vi "output_FPGA.vi"() -> ()   [LabVIEW 2021]
uses:
  <vilib>/Platform/TimedLoop/XDataNode/timing_clust.ctl
  <vilib>/Platform/TimedLoop/XDataNode/nitl_modes.ctl
  <vilib>/Platform/TimedLoop/XDataNode/wakeup.ctl
  <vilib>/rvi/Emulation/niFpgaGetClockAttributes.vi
  <vilib>/rvi/Emulation/niFpgaSctlEmulationGetInTimedLoop.vi
  <vilib>/rvi/Emulation/niFpgaEmulationReportErrorSimple.vi
  <vilib>/rvi/Emulation/niFpgaProcessEmulError.vi
  <vilib>/rvi/interface/RandomDataEmulation/niFpgaRandomDataHandleErrors.vi
  <vilib>/rvi/Emulation/niFpgaCriticalErrorInLSC.vi
  <vilib>/rvi/eio/common/nirviEmuTemplateMethod_errors.vi
  <vilib>/rvi/DataTransferAndStorage/Container/XNode/niFpgaContainer.xnode
  <vilib>/rvi/interface/RandomDataEmulation/nirviRandomDataFpgaReadWriteTemplate.vi
  <vilib>/eio/EIONode/EIONode.xnode
  <vilib>/Platform/TimedLoop/XDataNode/XDataNode.xnode
  <vilib>/Platform/TimedLoop/XDataNode/XDNodeRunTimeDep.lvlib
panel:
  out "Connector 1 DIO Port 0":u8
  out "Connector 1 DIO Port 1":u8
  out "Connector 1 DIO Port 2":u8
  out "Connector 1 DIO Port 3":u8
  in  "Connector 2 DIO Port 0":u8
  in  "Connector 2 DIO Port 1":u8
  out "AO: Actual Loop Rate(ticks)":u32
  in  "AO 0":i16
  in  "AO 1":i16
  in  "AO 2":i16
  in  "AO 3":i16
  in  "AO 4":i16
  in  "AO 5":i16
  in  "AO 6":i16
  in  "AO 7":i16
  in  "AO Loop Timer(Ticks)":u32
  out "AO Buffer Underflow?":bool
  in  "AO Buffer Enable":u8 format="%08b"
  in  "AO Enable":bool
  # "Analog Output"
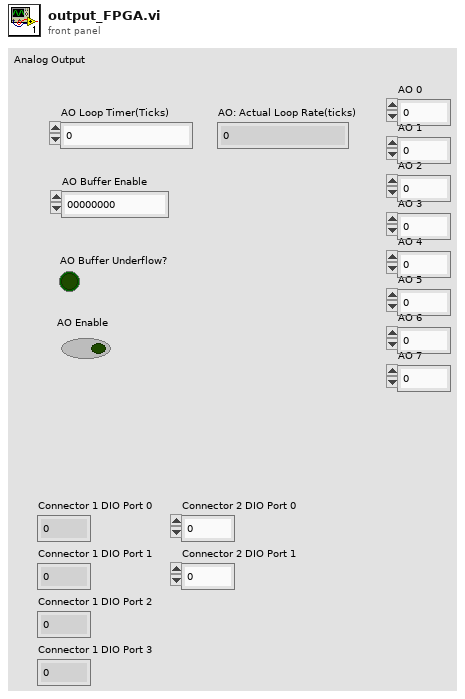
[diagram p1: front panel]
types:
  T1 = typedef "XDNodeRunTimeDep.lvlib/timing_clust.ctl" = cluster{"Expected End [f-1]":u64, "Actual End [f-1]":u64, "Finished Late? [f-1]":bool, "Expected End [i-1]":u64, "Actual End [i-1]":u64, "Finished Late? [i-1]":bool, "Expected Start [i]":u64, "Actual Start [i]":u64, "Expected Start [f]":u64, "Actual Start [f]":u64, "Source Name":string, "Structure Name":string, "Period":i64, "Deadline":i64, "Offset":i64, "Start":i64, "Priority":i32, "Timeout":i32, "Mode":T2, "Wakeup Reason":T3, "Error":errorcluster, "Source Type":string, "Secondary Source Type":string, "Global End Time":u64, "Global Start Time":u64, "Frame Duration":u64, "Iteration Duration":u64, "Assigned CPU":i32, "I/O Scan Engine Mode":u32}
  T2 = typedef "XDNodeRunTimeDep.lvlib/nitl_modes.ctl" = enum32{"No Change", "Process missed periods, maintain original phase", "Discard missed periods, maintain original phase", "Process missed periods, ignore original phase", "Discard missed periods, ignore original phase"}
  T3 = typedef "XDNodeRunTimeDep.lvlib/wakeup.ctl" = enum32{"Normal", "Aborted", "Asynchronous wakeup", "Timing source error", "Timed loop error", "Timeout"}
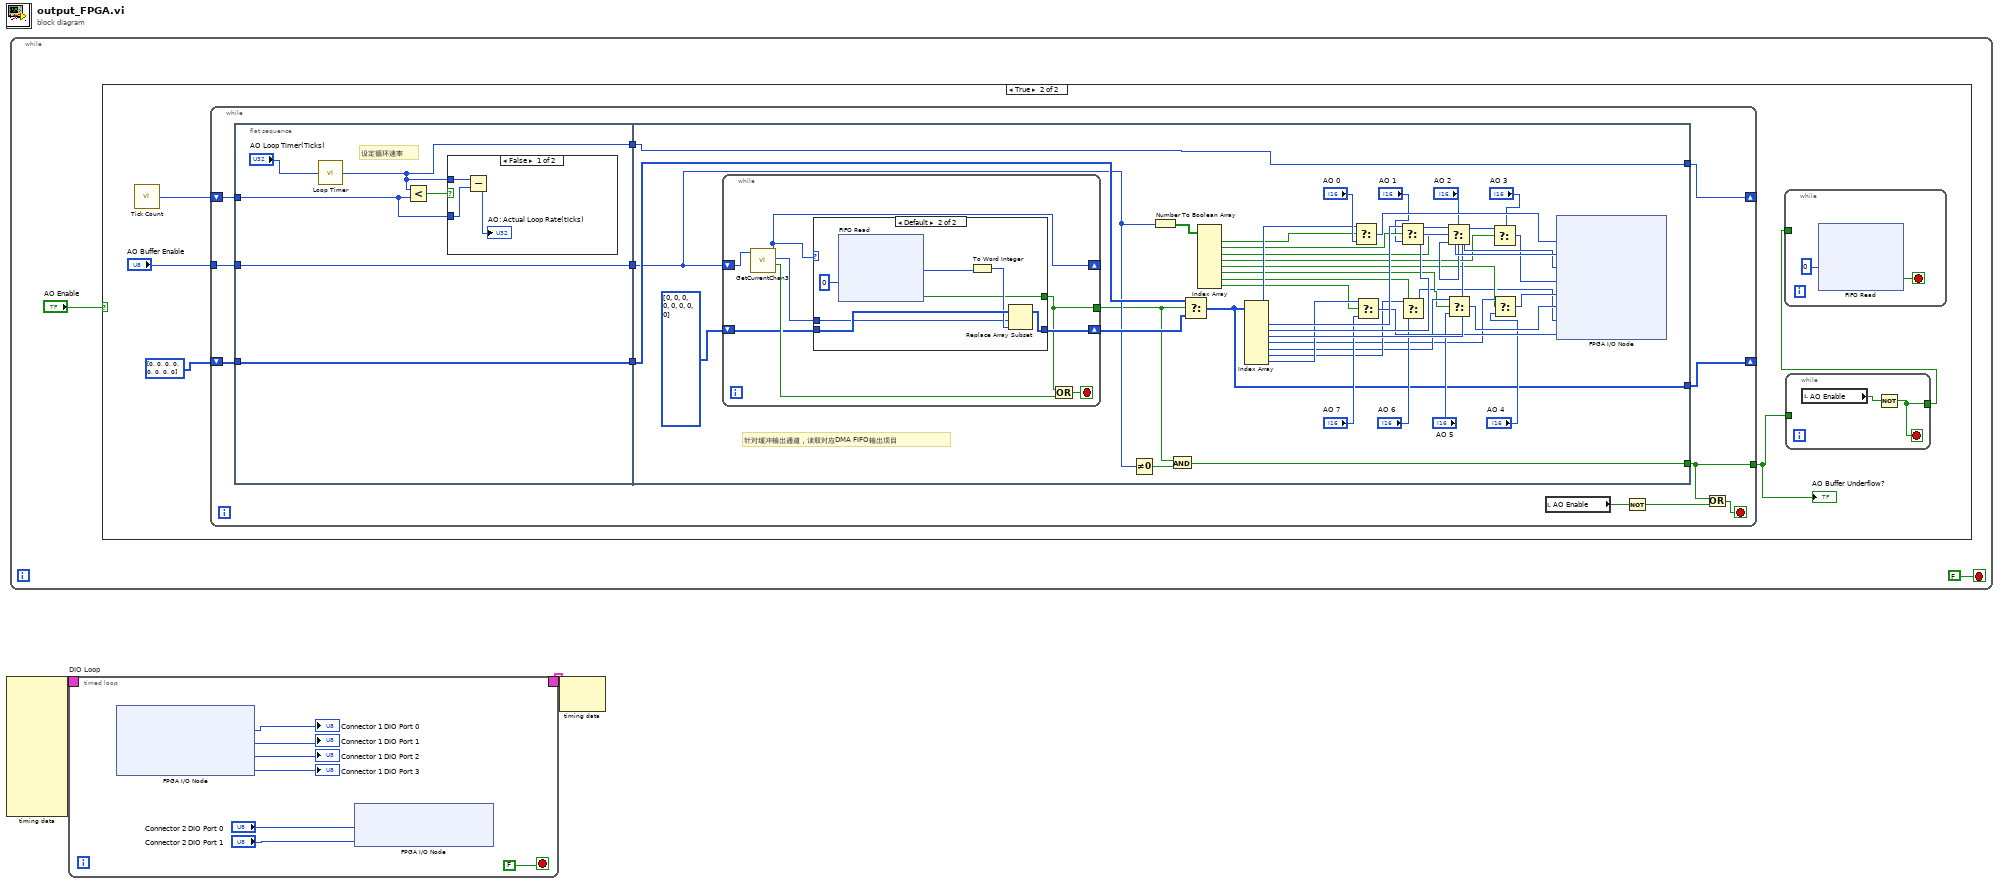
[diagram p0: block diagram]
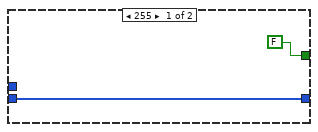
[diagram p4: hidden frame]
diagram:
  n1 = node-c288() -> (w2:T1)  [unwired: 10 in]
  n2 = while {
    stop <- FALSE stop-if-true
    n3 = case shown="True" "AO Enable" {
      frame False {
      }
      frame True {
        n4 = call "Tick Count"() -> ("Tick Count(Ticks)"=w9:u32)
        n5 = while {
          shift-right: [w14] -> _
          shift-left: w9 -> [w21]
          tunnel: "AO Buffer Enable" -> [w19]
          shift-right: [w15] -> _
          shift-left: i16[] [0, 0, 0, 0, 0, 0, 0, 0] -> [w16]
          tunnel: [w10] -> w6
          stop <- w12 stop-if-true
          n6 = flat-sequence {
            tunnel: w21 -> [w25]
            tunnel: [w24] -> w20
            tunnel: w19 -> [w24]
            tunnel: [w23] -> w18
            tunnel: [w22] -> w17
            tunnel: w16 -> [w22]
            tunnel: w20 -> [w67]
            tunnel: w18 -> [w33]
            tunnel: w17 -> [w70]
            tunnel: [w34] -> w15
            tunnel: [w33] -> w14
            tunnel: [w32] -> w10
            frame #0 {
              # "设定循环速率"
              n7 = call "Loop Timer"("Count(Ticks)"="AO Loop Timer(Ticks)") -> ("Tick Count(Ticks)"=w23:u32)
              n8 = Less?(x=w23, y=w25) -> (x < y?=w27:bool)
              n9 = case shown="False" w27 {
                tunnel: w23 -> [w30 _]
                tunnel: w25 -> [w29 _]
                frame False {
                  n10 = Subtract(x=w30, y=w29) -> (x-y=→"AO: Actual Loop Rate(ticks)":u32)
                }
                frame True {
                  # "overflow"
                }
              }
            }
            frame #1 {
              # "针对缓冲输出通道，读取对应DMA FIFO输出项目"
              n11 = while {
                shift-right: [w74] -> w71
                shift-left: i16[] [0, 0, 0, 0, 0, 0, 0, 0] -> [w78]
                shift-right: [w75] -> _
                shift-left: w67 -> [w76]
                tunnel: [w73] -> w66
                stop <- w79 stop-if-true
                n12 = call "GetCurrentChan3.vi"("AI Select In"=w76) -> ("Stop Loop"=w80:bool, "Current Channel"=w77:u8, "AI Select Out"=w75:u8)  [unwired: 8 in]
                n13 = case shown="Default" w75 {
                  tunnel: w78 -> [w81 w87]
                  tunnel: [w81 w86] -> w74
                  tunnel: [FALSE ("Empty") w83] -> w73
                  tunnel: w77 -> [_ w84]
                  frame 255 {
                  }
                  frame Default {
                    n14 = xnode ("FIFO Read")("Timeout"=0) -> ("Element"=w88:u32, "Timed Out?"=w83:bool)  [unwired: 1 in, 1 out]
                    n15 = To Word Integer(number=w88) -> (16bit integer=w85:i16)
                    n16 = Replace Array Subset(array=w87, new element=w85, index=w84) -> (w86:i16[])
                  }
                }
                n17 = Or(x=w73, y=w80) -> (x .or. y?=w79:bool)
              }
              n18 = Not Equal To 0?(x=w67) -> (x != 0?=w68:bool)
              n19 = Number To Boolean Array(number=w67) -> (Boolean array=w69:bool[])
              n20 = And(x=w66, y=w68) -> (x .and. y?=w32:bool)
              n21 = Select(t=w70, s=w66, f=w71) -> (s? t:f=w34:i16[])
              n22 = Index Array(array=w69) -> (element #1=w59:bool, element #2=w58:bool, element #3=w57:bool, element #4=w53:bool, element #5=w35:bool, element #6=w36:bool, element #7=w37:bool, element #8=w48:bool)  [unwired: 8 in]
              n23 = Index Array(array=w34) -> (element #1=w64:i16, element #2=w63:i16, element #3=w60:i16, element #4=w51:i16, element #5=w38:i16, element #6=w39:i16, element #7=w40:i16, element #8=w49:i16)  [unwired: 8 in]
              n24 = Select(t=w64, s=w59, f="AO 0") -> (s? t:f=w62:i16)
              n25 = Select(t=w49, s=w48, f="AO 7") -> (s? t:f=w46:i16)
              n26 = Select(t=w63, s=w58, f="AO 1") -> (s? t:f=w61:i16)
              n27 = Select(t=w40, s=w37, f="AO 6") -> (s? t:f=w31:i16)
              n28 = Select(t=w60, s=w57, f="AO 2") -> (s? t:f=w54:i16)
              n29 = Select(t=w39, s=w36, f="AO 5") -> (s? t:f=w43:i16)
              n30 = Select(t=w51, s=w53, f="AO 3") -> (s? t:f=w50:i16)
              n31 = Select(t=w38, s=w35, f="AO 4") -> (s? t:f=w41:i16)
              n32 = xnode "FPGA I/O Node"("Connector0/AO0"=w62, "Connector0/AO1"=w61, "Connector0/AO2"=w54, "Connector0/AO3"=w50, "Connector0/AO4"=w41, "Connector0/AO5"=w43, "Connector0/AO6"=w31, "Connector0/AO7"=w46) -> ()  [unwired: 8 in, 8 out]
            }
          }
          n33 = local read "AO Enable"() -> (w11:bool)
          n34 = Not(x=w11) -> (.not. x?=w13:bool)
          n35 = Or(x=w10, y=w13) -> (x .or. y?=w12:bool)
        }
        "AO Buffer Underflow?" <- w6
        n36 = while {
          tunnel: w6 -> [_]
          tunnel: [w92] -> w5
          stop <- w92 stop-if-true
          n37 = local read "AO Enable"() -> (w93:bool)
          n38 = Not(x=w93) -> (.not. x?=w92:bool)
        }
        n39 = while {
          tunnel: w5 -> [_]
          stop <- w90 stop-if-true
          n40 = xnode ("FIFO Read")("Timeout"=0) -> ("Timed Out?"=w90:bool)  [unwired: 1 in, 2 out]
        }
      }
    }
  }
  n41 = timed-loop "DIO Loop" {
    timing: w2 -> [_]
    timing-out: [_] -> w1
    stop <- FALSE stop-if-true
    n42 = xnode "FPGA I/O Node"() -> ("Connector1/DIOPORT0"=→"Connector 1 DIO Port 0":u8, "Connector1/DIOPORT1"=→"Connector 1 DIO Port 1":u8, "Connector1/DIOPORT2"=→"Connector 1 DIO Port 2":u8, "Connector1/DIOPORT3"=→"Connector 1 DIO Port 3":u8)  [unwired: 4 in, 4 out]
    n43 = xnode "FPGA I/O Node"("Connector0/DIOPORT0"="Connector 2 DIO Port 0", "Connector0/DIOPORT1"="Connector 2 DIO Port 1") -> ()  [unwired: 2 in, 2 out]
  }
  n44 = node-c288(w1) -> ()  [unwired: 1 out]
